vi "Send Reinitialize All Msg.vi"(10 "Mode":string, 11 "Message Enqueuer in":refnum<class "Message Enqueuer.lvclass">) -> (3 "Message Enqueuer out":refnum<class "Message Enqueuer.lvclass">)   [LabVIEW 2013, in "Abstract Messages.lvlib"]
uses:
  <vilib>/ActorFramework/Message Enqueuer/Message Enqueuer.lvclass
  Abstract Reinitialize All Msg.lvclass
  <vilib>/ActorFramework/Message Enqueuer/Message Enqueuer.lvclass/Message Enqueuer.ctl
  <vilib>/ActorFramework/Message Priority Queue/Priority Enqueue.vi
  Abstract Messages.lvlib
  <vilib>/ActorFrameworkMVC/UI Controller Messages/Get Model Actor Enqueuer Msg/Get Model Actor Enqueuer Msg.lvclass
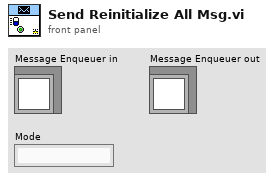
[diagram p1: front panel]
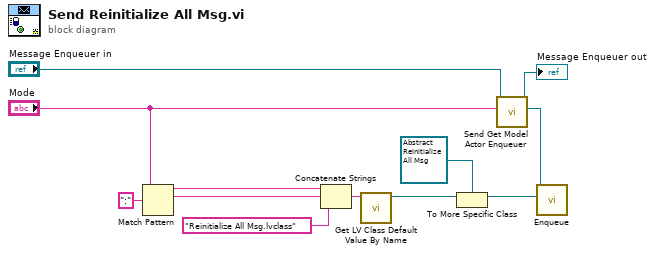
[diagram p0: block diagram]
diagram:
  n1 = Match Pattern(string="Mode", regular expression=":") -> (before substring=w8:string, match substring=w9:string)  [unwired: 1 in, 2 out]
  n2 = Concatenate Strings(w8, w9, "Reinitialize All Msg.lvclass" ("element")) -> (w10:string)
  n3 = call <vilib>:"Get LV Class Default Value By Name.vi"("class name"=w10) -> ("object"=w6:refnum<class>)  [unwired: 9 in, 1 out]
  n4 = To More Specific Class(target class=refnum<class "Abstract Reinitialize All Msg.lvclass"> refnum ("Abstract Messages.lvlib:Abstract Reinitialize All Msg.lvclass"), reference=w6) -> (specific class reference=w11:refnum<class "Abstract Reinitialize All Msg.lvclass">)  [unwired: 1 in, 1 out]
  n5 = call <vilib>:"Send Get Model Actor Enqueuer.vi"("Model Name"="Mode", "Message Enqueuer in"="Message Enqueuer in") -> ("Reply"=w1:refnum<class "Message Enqueuer.lvclass">, "Message Enqueuer out"=→"Message Enqueuer out":refnum<class "Message Enqueuer.lvclass">)  [unwired: 6 in, 2 out]
  n6 = call <vilib>:"Enqueue.vi"("Message"=w11, "Message Enqueuer in"=w1) -> ()  [unwired: 8 in, 2 out]
